vi "Right-Click Target.vi"(10 "State In":T2={"Worker Library Path"=path "", "Block Label"="", "Types"=[], "Selections"=[], "Icon"={"image type"=0, "image depth"=0, "image"=[], "mask"=[], "colors"=[], "Rectangle"={"left"=0, "top"=0, "right"=0, "bottom"=0}}, "Errors"={"Terminals"=[], "Generate"={"status"=FALSE, "code"=0, "source"=""}, "General"={"status"=FALSE, "code"=0, "source"=""}}, "Calculated Sizes"={"Block Width"=0, "Block Height"=0, "Half Width"=0, "Icon Top"=0, "Icon Bottom"=0, "Label Width"=0, "Half Label"=0, "Label Top"=0, "Text Width"=0, "Half Text"=0, "Text Height"=0, "Label Height"=0, "Expanded Width"=0, "Label Bottom"=0, "Expanded Top"=0, "Expanded Bottom"=0, "Expanded Height"=0, "Min Height"=0, "Max Height"=0}, "Special Terminal Indices"={"Action"=-1, "Init"=-1, "Tag"=-1, "State in"=-1, "State out"=-1, "Error"=-1, "Control"=-1, "Config"=-1}, "Terminals"=[], "Temp VI Name"="", "Description"="", "Smol Mode"=FALSE}, 11 "Point":T14) -> (1 "Target Index":i32, 3 "Menu Target":T1)   [LabVIEW 2022 SP3, in "FlexBlocks Support.lvlib"]
uses:
  FlexBlocks Support.lvlib
  Right-Click Menu Target.ctl
  <vilib>/XNodeSupport/XNodeInt.ctl
  <vilib>/XNodeSupport/NI_XNodeSupport.lvlib
  <vilib>/XNodeSupport/XNodePoint.ctl
  Terminal Direction.ctl
  Value Mode.ctl
  Special Terminal.ctl
  Type Descriptor.ctl
  <vilib>/picture/picture.llb/imagedata.ctl
  XNode Errors.ctl
  Calculated Sizes.ctl
  Special Terminal Indices.ctl
  Terminal State.ctl
  Terminal Draw Style.ctl
  Terminal Status.ctl
  Flex Block/State.ctl
  Flex Block/Flex Block.xnode
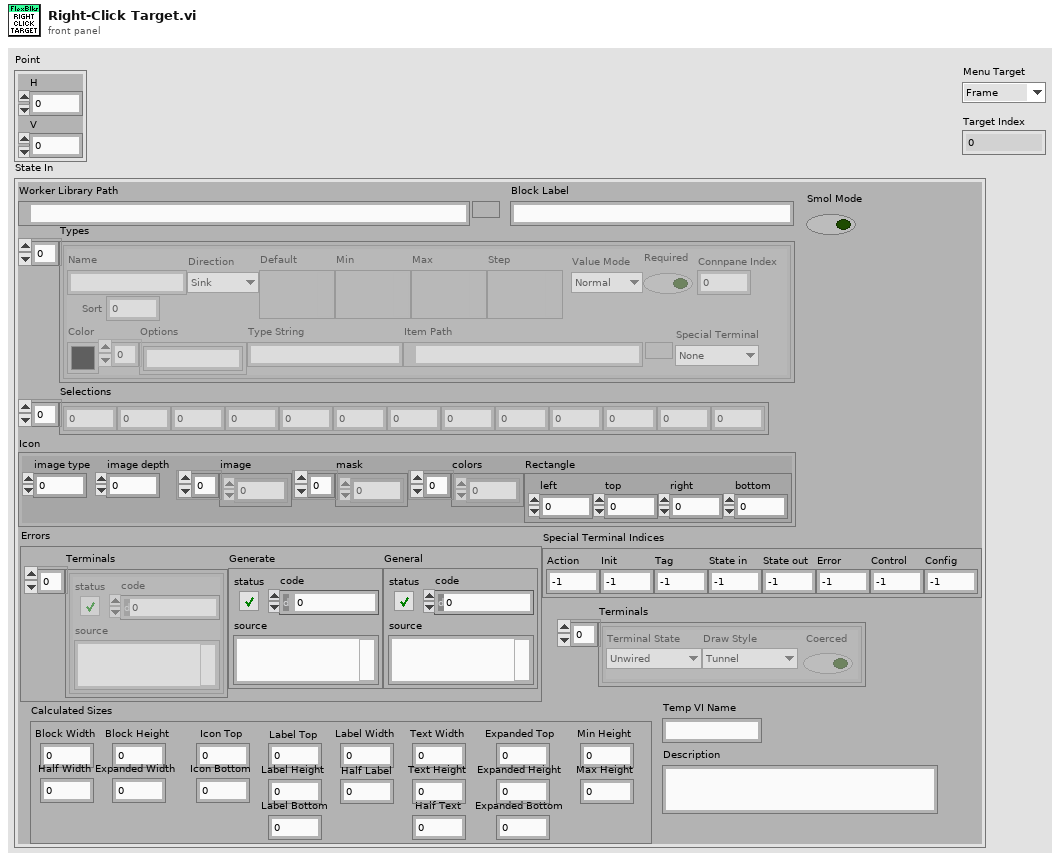
[diagram p1: front panel]
types:
  T1 = typedef "FlexBlocks Support.lvlib/Right-Click Menu Target.ctl" = enum16{"Frame", "Label", "Value", "Terminal", "Icon"}
  T2 = typedef "Flex Block.xnode/State.ctl" = cluster{"Worker Library Path":path, "Block Label":string, "Types":T3[], "Selections":i32[], "Icon":T7, "Errors":T8, "Calculated Sizes":T9, "Special Terminal Indices":T10, "Terminals":T11[], "Temp VI Name":string, "Description":string, "Smol Mode":bool}
  T3 = typedef "FlexBlocks Support.lvlib/Type Descriptor.ctl" = cluster{"Name":string, "Direction":T4, "Default":variant, "Min":variant, "Max":variant, "Step":variant, "Value Mode":T5, "Color":u32, "Options":string[], "Type String":string, "Item Path":path, "Required":bool, "Connpane Index":i32, "Special Terminal":T6, "Sort":i32}
  T4 = typedef "FlexBlocks Support.lvlib/Terminal Direction.ctl" = enum16{"Sink", "Source"}
  T5 = typedef "FlexBlocks Support.lvlib/Value Mode.ctl" = enum16{"Normal", "Range", "Select"}
  T6 = typedef "FlexBlocks Support.lvlib/Special Terminal.ctl" = enum16{"None", "Action", "Init", "Tag", "State in", "State out", "Error", "Control", "Config"}
  T7 = typedef "imagedata.ctl" = cluster{"image type":i32, "image depth":i32, "image":u8[], "mask":u8[], "colors":u32[], "Rectangle":cluster{"left":i16, "top":i16, "right":i16, "bottom":i16}}
  T8 = typedef "FlexBlocks Support.lvlib/XNode Errors.ctl" = cluster{"Terminals":errorcluster[], "Generate":errorcluster, "General":errorcluster}
  T9 = typedef "FlexBlocks Support.lvlib/Calculated Sizes.ctl" = cluster{"Block Width":i32, "Block Height":i32, "Half Width":i32, "Icon Top":i32, "Icon Bottom":i32, "Label Width":i32, "Half Label":i32, "Label Top":i32, "Text Width":i32, "Half Text":i32, "Text Height":i32, "Label Height":i32, "Expanded Width":i32, "Label Bottom":i32, "Expanded Top":i32, "Expanded Bottom":i32, "Expanded Height":i32, "Min Height":i32, "Max Height":i32}
  T10 = typedef "FlexBlocks Support.lvlib/Special Terminal Indices.ctl" = cluster{"Action":i32, "Init":i32, "Tag":i32, "State in":i32, "State out":i32, "Error":i32, "Control":i32, "Config":i32}
  T11 = typedef "FlexBlocks Support.lvlib/Terminal Status.ctl" = cluster{"Terminal State":T12, "Draw Style":T13, "Coerced":bool}
  T12 = typedef "FlexBlocks Support.lvlib/Terminal State.ctl" = enum16{"Unwired", "BadType", "BadRef", "Channel", "Value", "Control Ref"}
  T13 = typedef "FlexBlocks Support.lvlib/Terminal Draw Style.ctl" = enum16{"Tunnel", "BadType", "BadRef", "Channel", "Value", "Control Ref"}
  T14 = typedef "NI_XNodeSupport.lvlib/XNodePoint.ctl" = cluster{"H":T15, "V":T15}
  T15 = typedef "NI_XNodeSupport.lvlib/XNodeInt.ctl" = i32
  T16 = typedef "FlexBlocks Support.lvlib/Size Constants.ctl" = cluster{"Icon Size":i32, "Name H Pad":i32, "Name V Pad":i32, "Max Label Width":i32, "Value Width":i32, "Frame Padding":i32, "Vertical Margin":i32, "Min Width":i32, "Min Height":i32, "Collapsed Spacing":i32, "Terminal Center Offset":i32}
  T17 = cluster{"Icon Top":i32, i32, "Icon Bottom":i32, i32}
  T18 = cluster{"Expanded Top":i32, "Frame Padding":i32, "Expanded Bottom":i32, i32}
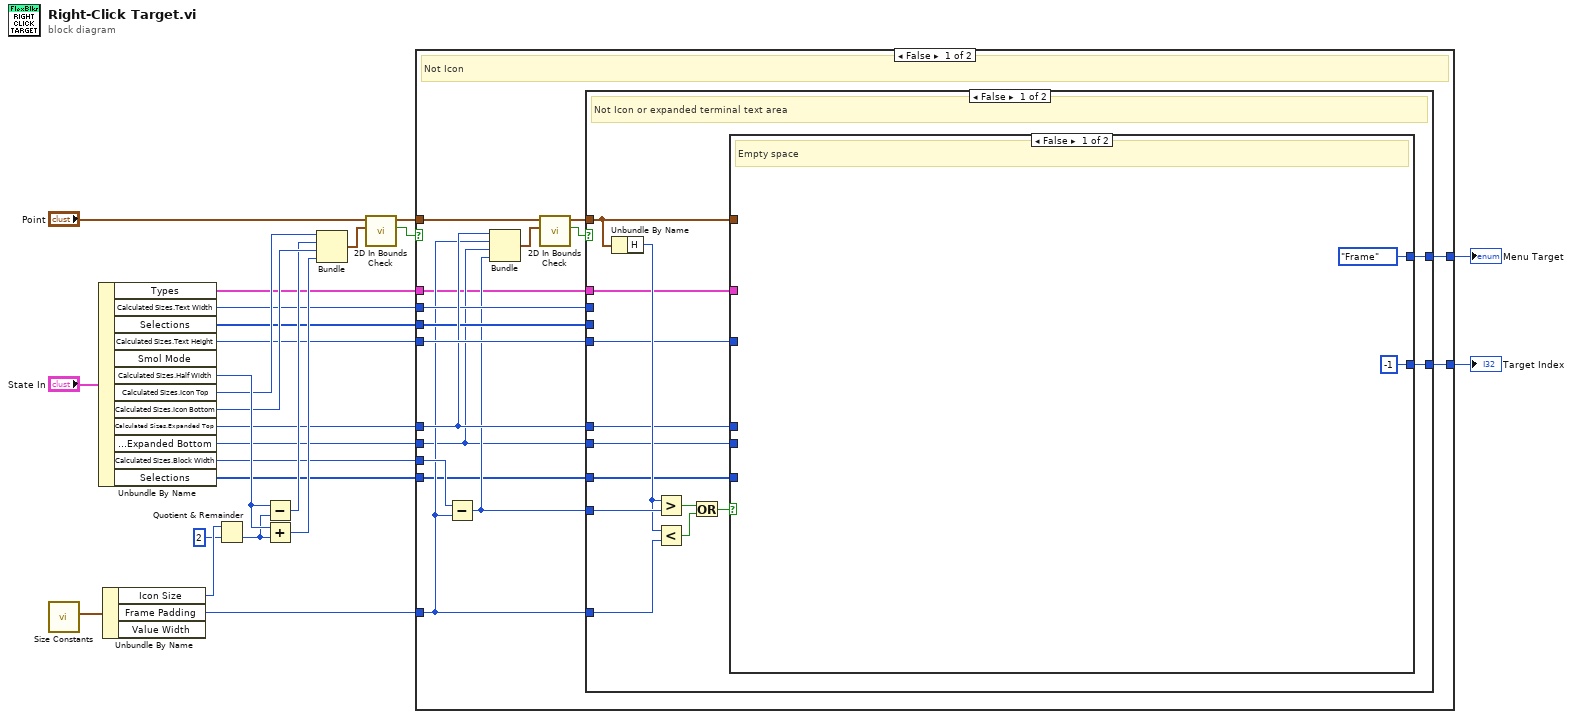
[diagram p0: block diagram]
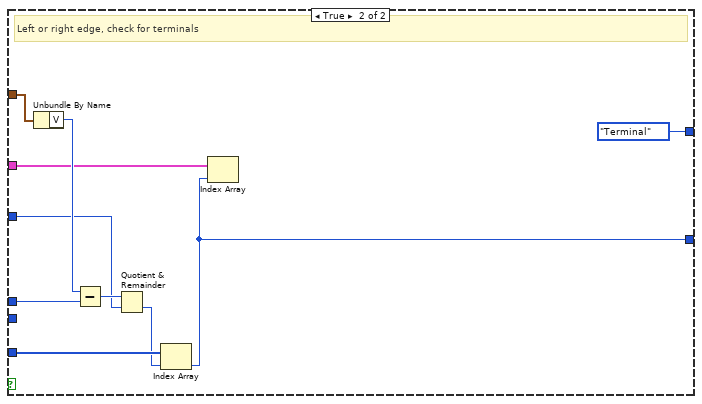
[diagram p2: hidden frame]
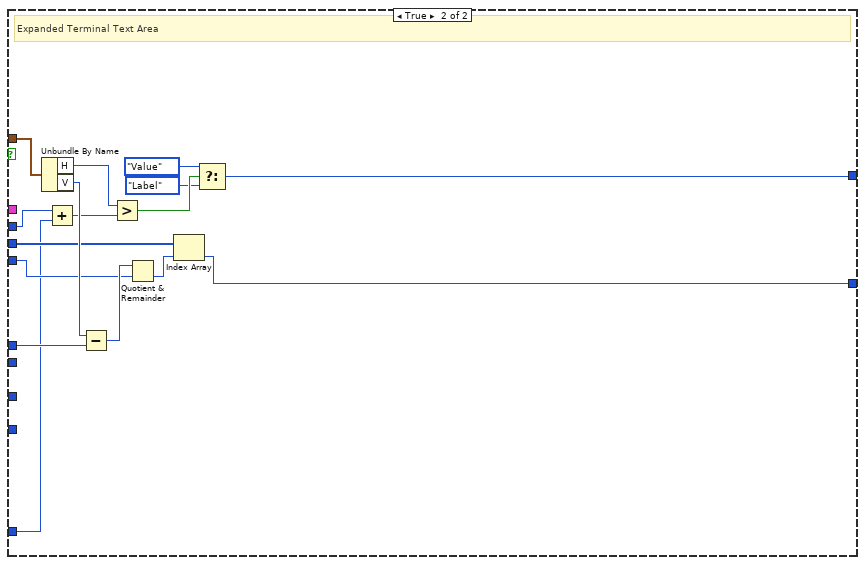
[diagram p3: hidden frame]
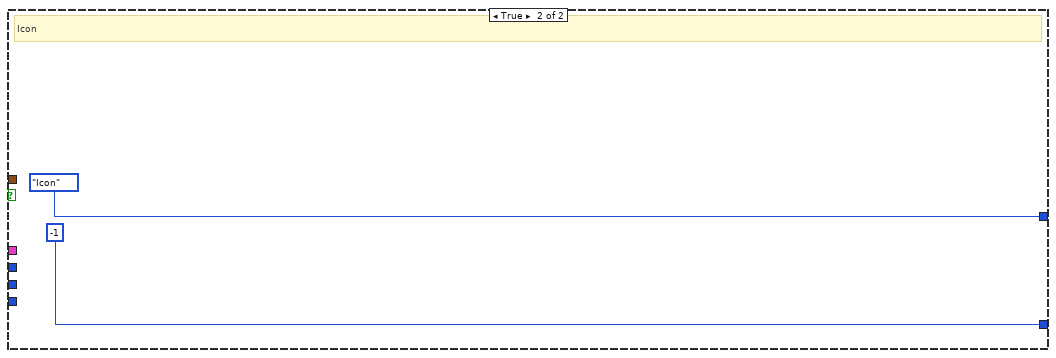
[diagram p4: hidden frame]
diagram:
  n1 = call "Size Constants.vi"() -> ("Size Constants"=w24:T16)  [unwired: 11 in]
  n2 = Unbundle By Name("State In") -> ("Types"=w2:T3[], "Calculated Sizes.Text Width"=w3:i32, "Selections"=w4:i32[], "Calculated Sizes.Text Height"=w5:i32, "Calculated Sizes.Half Width"=w21:i32, "Calculated Sizes.Icon Top"=w19:i32, "Calculated Sizes.Icon Bottom"=w18:i32, "Calculated Sizes.Expanded Top"=w9:i32, "Calculated Sizes.Expanded Bottom"=w8:i32, "Calculated Sizes.Block Width"=w7:i32, "Selections"=w1:i32[])  [unwired: 1 out]
  n3 = Unbundle By Name(w24) -> ("Icon Size"=w23:i32, "Frame Padding"=w6:i32)  [unwired: 1 out]
  n4 = Quotient & Remainder(x=w23, y=2) -> (floor(x/y)=w20:i32)  [unwired: 1 out]
  n5 = Subtract(x=w21, y=w20) -> (x-y=w17:i32)
  n6 = Add(x=w21, y=w20) -> (x+y=w16:i32)
  n7 = Bundle("Icon Top"=w19, w17, "Icon Bottom"=w18, w16) -> (w14:T17)  [unwired: 1 in]
  n8 = call "2D In Bounds Check.vi"("Bounds"=w14, "Point in"="Point") -> ("In Bounds?"=w13:bool, "Point"=w12:cluster{"H":T15, "V":T15})  [unwired: 8 in]
  n9 = case shown="False" w13 {
    tunnel: w12 -> [w41 _]
    tunnel: [w36 Right-Click_Menu_Target."Icon" ("Menu Target")] -> w11
    tunnel: [w32 -1 ("Index")] -> w10
    tunnel: w9 -> [w34 _]
    tunnel: w8 -> [w28 _]
    tunnel: w7 -> [w40 _]
    tunnel: w6 -> [w30 _]
    tunnel: w5 -> [w35 _]
    tunnel: w4 -> [w33 _]
    tunnel: w3 -> [w31 _]
    tunnel: w2 -> [w27 _]
    tunnel: w1 -> [w26 _]
    frame False {
      # "Not Icon"
      n10 = Subtract(x=w40, y=w30) -> (x-y=w29:i32)
      n11 = Bundle("Expanded Top"=w34, "Frame Padding"=w30, "Expanded Bottom"=w28, w29) -> (w39:T18)  [unwired: 1 in]
      n12 = call "2D In Bounds Check.vi"("Bounds"=w39, "Point in"=w41) -> ("In Bounds?"=w37:bool, "Point"=w38:cluster{"H":T15, "V":T15})  [unwired: 8 in]
      n13 = case shown="False" w37 {
        tunnel: w38 -> [w49 w83]
        tunnel: [w43 w69] -> w36
        tunnel: w35 -> [w46 w79]
        tunnel: w34 -> [w48 w82]
        tunnel: w33 -> [_ w78]
        tunnel: [w42 w76] -> w32
        tunnel: w31 -> [_ w75]
        tunnel: w30 -> [w54 w74]
        tunnel: w29 -> [w55 _]
        tunnel: w28 -> [w47 _]
        tunnel: w27 -> [w45 _]
        tunnel: w26 -> [w44 _]
        frame False {
          # "Not Icon or expanded terminal text area"
          n14 = Unbundle By Name(w49) -> ("H"=w53:T15)
          n15 = Greater?(x=w53, y=w55) -> (0:w52:bool)
          n16 = Less?(x=w53, y=w54) -> (x < y?=w51:bool)
          n17 = Or(x=w52, y=w51) -> (x .or. y?=w50:bool)
          n18 = case shown="False" w50 {
            tunnel: w49 -> [_ w67]
            tunnel: w48 -> [_ w66]
            tunnel: w47 -> [_ _]
            tunnel: w46 -> [_ w63]
            tunnel: w45 -> [_ w60]
            tunnel: w44 -> [_ w62]
            tunnel: [Right-Click_Menu_Target."Frame" ("Menu Target") Right-Click_Menu_Target."Terminal" ("Menu Target")] -> w43
            tunnel: [-1 ("Numeric") w58] -> w42
            frame False {
              # "Empty space"
            }
            frame True {
              # "Left or right edge, check for terminals"
              n19 = Unbundle By Name(w67) -> ("V"=w65:T15)
              n20 = Subtract(x=w65, y=w66) -> (x-y=w64:T15)
              n21 = Quotient & Remainder(x=w64, y=w63) -> (floor(x/y)=w61:T15)  [unwired: 1 out]
              n22 = Index Array(array=w62, index=w61) -> (element=w58:i32)
              n23 = Index Array(array=w60, index=w58) -> ()  [unwired: 1 out]
            }
          }
        }
        frame True {
          # "Expanded Terminal Text Area"
          n24 = Unbundle By Name(w83) -> ("H"=w72:T15, "V"=w81:T15)
          n25 = Add(x=w75, y=w74) -> (x+y=w73:i32)
          n26 = Subtract(x=w81, y=w82) -> (x-y=w80:T15)
          n27 = Greater?(x=w72, y=w73) -> (0:w71:bool)
          n28 = Quotient & Remainder(x=w80, y=w79) -> (floor(x/y)=w77:T15)  [unwired: 1 out]
          n29 = Index Array(array=w78, index=w77) -> (element=w76:i32)
          n30 = Select(t=Right-Click_Menu_Target."Value", s=w71, f=Right-Click_Menu_Target."Label" ("Menu Target")) -> (s? t:f=w69:T1)
        }
      }
    }
    frame True {
      # "Icon"
    }
  }
  "Menu Target" <- w11
  "Target Index" <- w10
